vi "kmakise.vi"() -> ()   [LabVIEW 2020]
uses:
  <vilib>/Instr/_visa.llb/VISA Configure Serial Port (Instr).vi
panel:
  out "接收数据":string
  out "序号":dbl(knob) scale=0.0..255.0
  out "波形图":dbl[](graph)
  out "通道 2":dbl[](array[numeric])
  out "ADC值":string[](array[string])
  out "电压mV":dbl[](array[numeric])
  in  "Enable Termination\nChar (T)":bool=TRUE caption="启用终止符 (T)"
  out "ARR[263]":u8
  in  "停止":bool
  out "VISA resource \nname out":refnum<visa-resource-name> caption="VISA资源名称输出"
  out "error out":errorcluster caption="错误输出"
  out "termination char\n(0xA = '\\n' = LF)":u8=10 caption="终止符\n(0xA = '\\n' = LF)" format="%.0x"
  in  "timeout (10sec)":u32=10000 caption="超时（10秒）"
  in  "flow control (0:none)":u16(ring) caption="流控制（0:无）" items=["无", "XON/XOFF", "RTS/CTS", "XON/XOFF & RTS/CTS", "DTR/DSR", "XON/XOFF & DTR/DSR"]
  in  "stop bits (10: 1 bit)":u16(ring)=10 caption="停止位（10: 1位）" items=["1.0"=10, "1.5"=15, "2.0"=20]
  in  "error in (no error)":errorcluster caption="错误输入（无错误）"
  in  "parity (0:none)":enum16{"None", "Odd", "Even", "Mark", "Space"}(ring) caption="奇偶（0:无）"
  in  "data bits (8)":u16=8 caption="数据比特(8)" min=5 max=8 step=1
  out "baud rate (9600)":u32=9600 caption="波特率(9600)"
  in  "VISA resource name":refnum<visa-resource-name> caption="VISA资源名称"
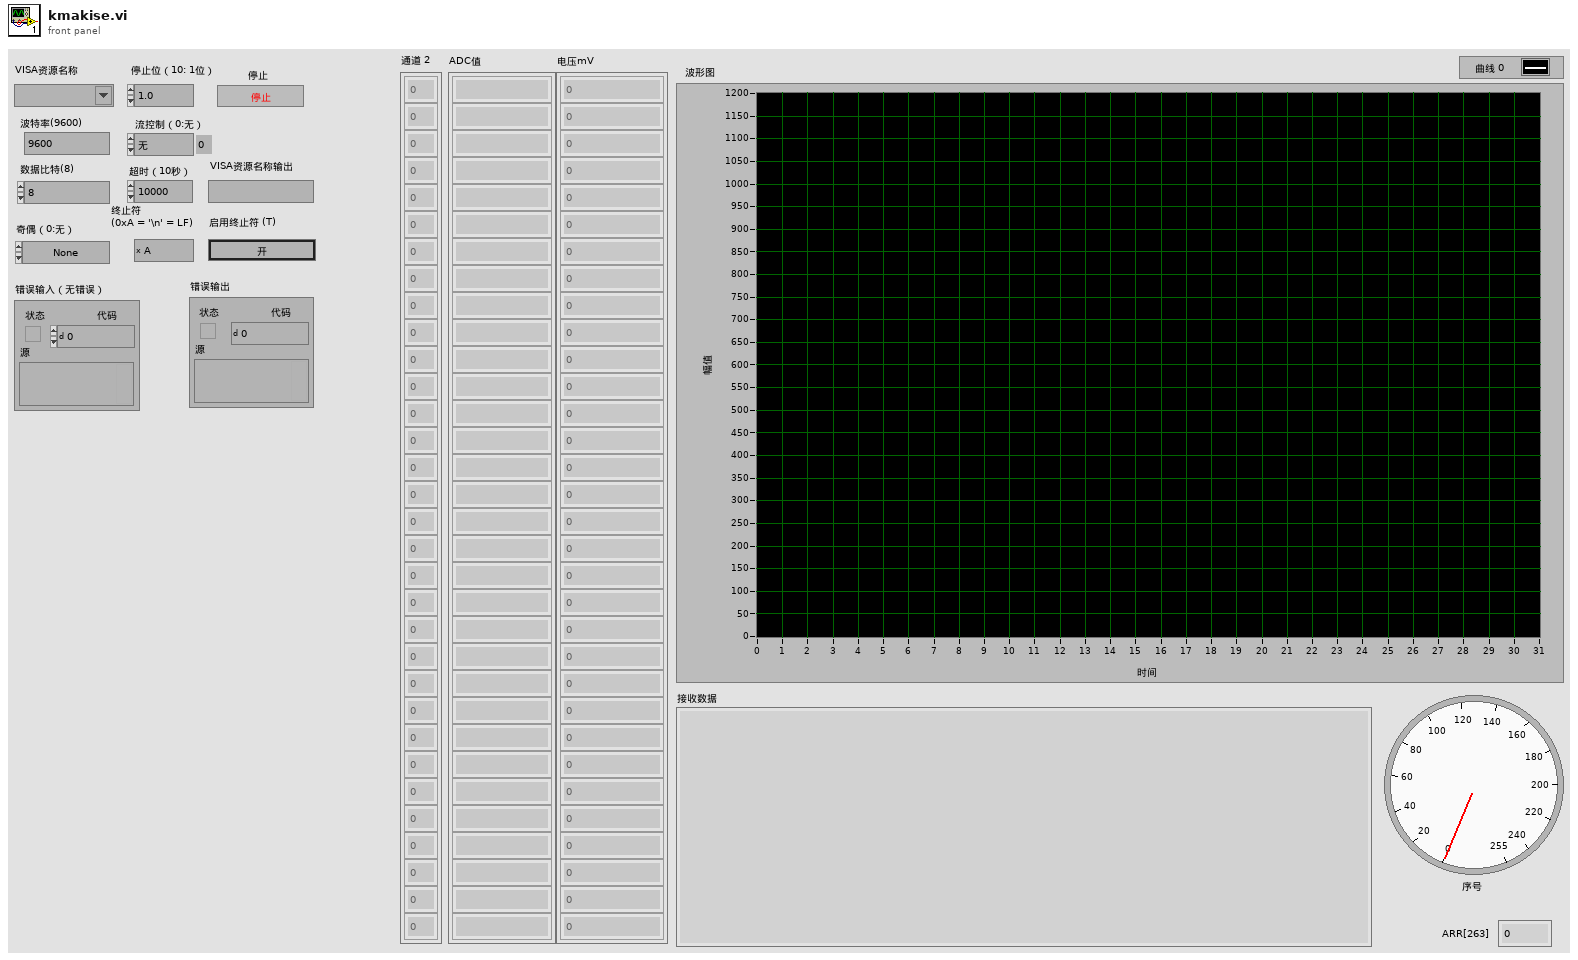
[diagram p1: front panel]
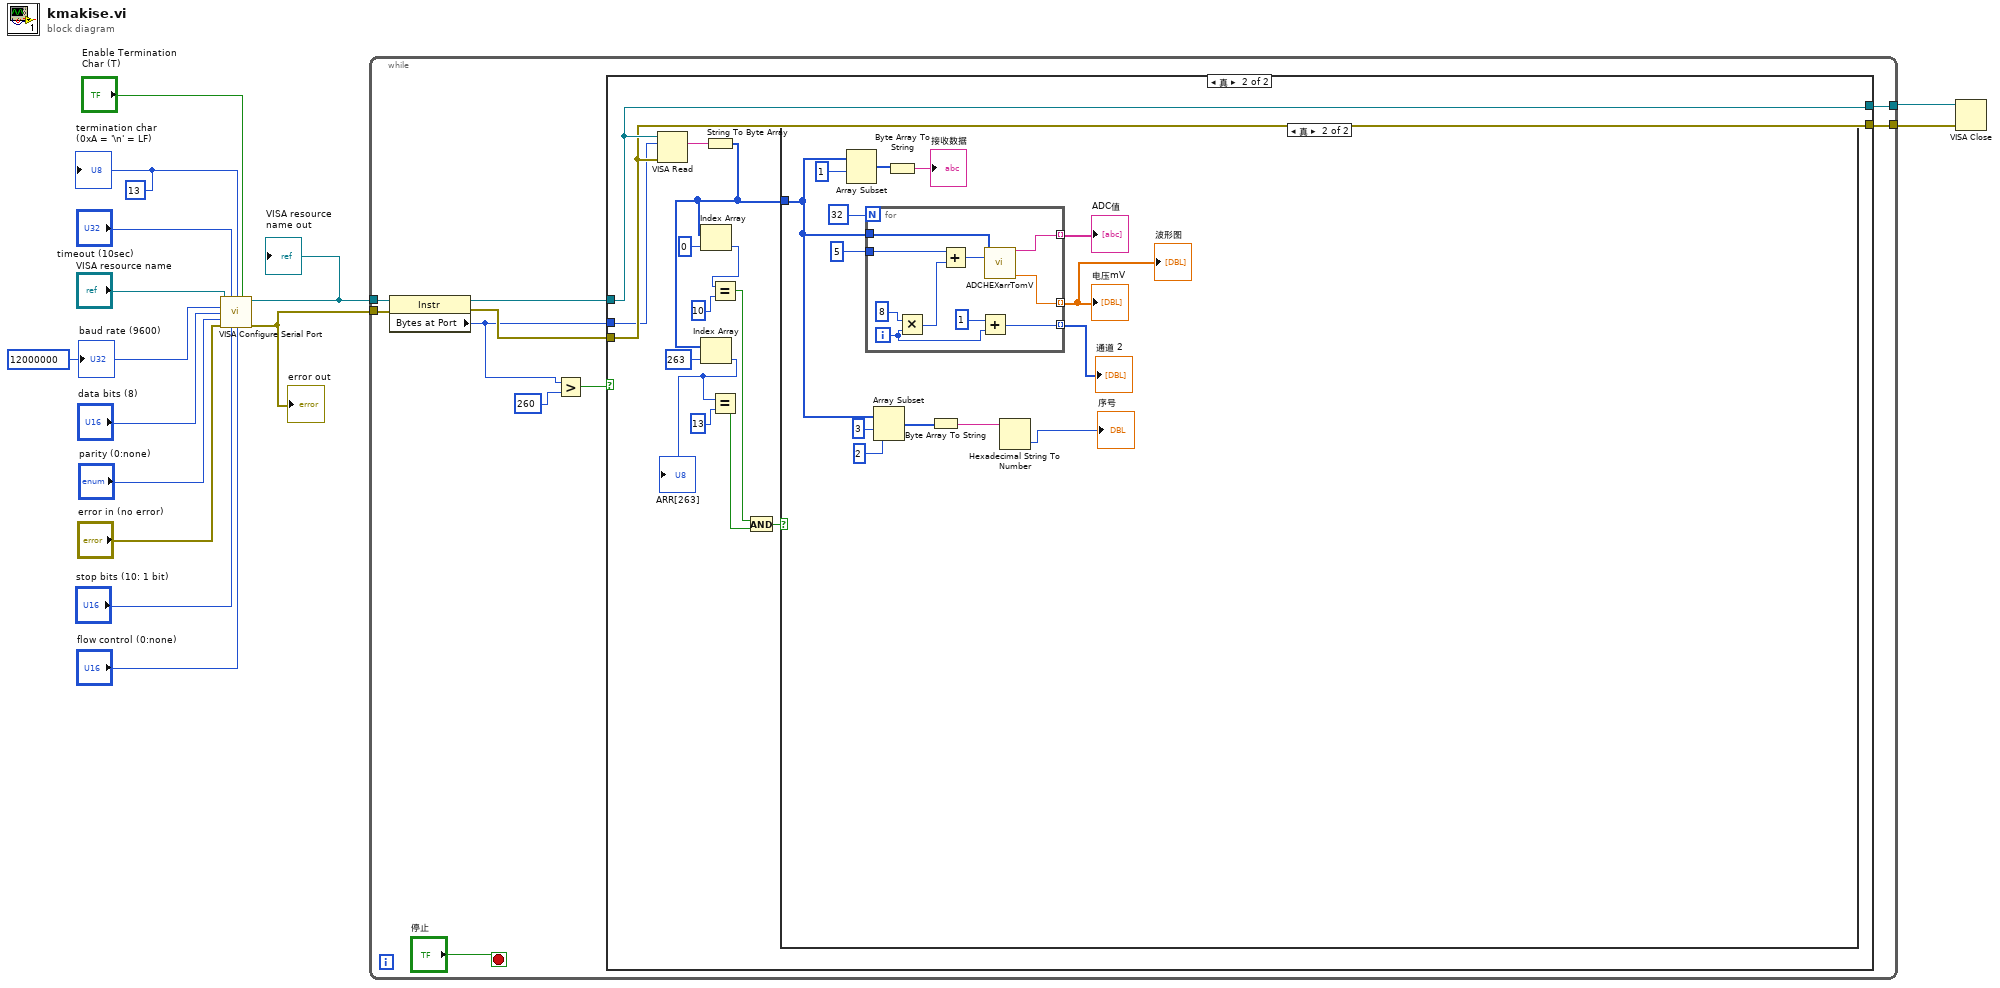
[diagram p0: block diagram]
diagram:
  w1 = u8 13 ("termination char\n(0xA = '\\n' = LF)")
  w3 = u32 12000000 ("baud rate (9600)")
  n1 = call-poly "VISA Configure Serial Port"("VISA resource name"="VISA resource name", "timeout (10sec)"="timeout (10sec)", "termination char\n(0xA = '\\n' = LF)"=w1, "Enable Termination\nChar (T)"="Enable Termination\nChar (T)", "baud rate (9600)"=w3, "data bits (8)"="data bits (8)", "parity (0:none)"="parity (0:none)", "error in (no error)"="error in (no error)", "stop bits (10: 1 bit)"="stop bits (10: 1 bit)", "flow control (0:none)"="flow control (0:none)") -> ("VISA resource name out"=w7:refnum<visa-resource-name>, "error out"=w6:errorcluster)  [unwired: 4 in]
  "error out" <- w6
  "VISA resource \nname out" <- w7
  n2 = while {
    tunnel: w7 -> [w24]
    tunnel: w6 -> [w23]
    tunnel: [w22] -> w5
    tunnel: [w21] -> w4
    stop <- "停止" stop-if-true
    n3 = property on="属性节点" class="Instr"(reference=w24, error in=w23) -> (reference out=w20:refnum<visa-resource-name>, error out=w19:errorcluster, "Bytes at Port"=w15:u32)
    n4 = Greater?(x=w15, y=u32 260) -> (0:w16:bool)
    n5 = case shown="真" w16 {
      tunnel: w15 -> [_ w30]
      tunnel: w20 -> [w26 w40]
      tunnel: w19 -> [w25 w39]
      tunnel: [w26 w40] -> w22
      tunnel: [w25 w39] -> w21
      frame False {
      }
      frame True {
        n6 = VISA Read(VISA resource name=w40, byte count=w30, error in (no error)=w39) -> (read buffer=w35:string)  [unwired: 3 out]
        n7 = String To Byte Array(string=w35) -> (unsigned byte array=w31:u8[])
        n8 = Index Array(array=w31, index=0 ("索引")) -> (element=w36:u8)
        n9 = Index Array(array=w31, index=263 ("索引")) -> (element=w32:u8)
        "ARR[263]" <- w32
        n10 = Equal?(x=w36, y=u8 10) -> (x = y?=w28:bool)
        n11 = Equal?(x=w32, y=u8 13) -> (x = y?=w27:bool)
        n12 = And(x=w28, y=w27) -> (x .and. y?=w29:bool)
        n13 = case shown="真" w29 {
          tunnel: w31 -> [_ w42]
          frame False {
          }
          frame True {
            n14 = Array Subset(array=w42, index=1 ("索引")) -> (w43:u8[])  [unwired: 1 in]
            n15 = for {
              N: 32 -> [_]
              tunnel: w42 -> [w64]
              tunnel: 5 ("索引") -> [w63]
              tunnel: [w59] -> w50 mode=indexing
              tunnel: [w58] -> w52 mode=indexing
              tunnel: [w57] -> w51 mode=indexing
              i -> [w56]
              n16 = Multiply(x=8 ("y"), y=w56) -> (x*y=w62:i32)
              n17 = Add(x=w63, y=w62) -> (x+y=w61:i32)
              n18 = Add(x=1, y=w56) -> (x+y=w57:i32)
              n19 = call "ADCHEXarrTomV.vi"("数组"=w64, "索引"=w61) -> ("ADC值"=w58:string, "电压mV"=w59:dbl)  [unwired: 11 in, 1 out]
            }
            "电压mV" <- w50
            "ADC值" <- w52
            "通道 2" <- w51
            "波形图" <- w50
            n20 = Array Subset(array=w42, index=3 ("索引"), length=2 ("长度")) -> (w49:u8[])
            n21 = Byte Array To String(unsigned byte array=w43) -> (string=→"接收数据":string)
            n22 = Byte Array To String(unsigned byte array=w49) -> (string=w46:string)
            n23 = Hexadecimal String To Number(string=w46) -> (number=→"序号":u32)  [unwired: 2 in, 1 out]
          }
        }
      }
    }
  }
  n24 = VISA Close(VISA resource name=w5, error in (no error)=w4) -> ()  [unwired: 1 out]
  "baud rate (9600)" <- w3
  "termination char\n(0xA = '\\n' = LF)" <- w1
